vi "Calculate_Error_Rate.vi"(6 "Dataset(In1D_Out1D)":T1, 11 "Predictions":sgl[][](array[numeric])) -> (3 "Numeric":dbl)   [LabVIEW 2020]
uses:
  <vilib>/Ngene/DeepLTK/Toolkit/NN_Data/API/DataSet_Types/NN_DataSet(In1D_Out1D).ctl
  <vilib>/Ngene/DeepLTK/Toolkit/NN_Data/API/DataRef_Types/NN_Data_ref(2D_SGL).ctl
  <vilib>/Ngene/DeepLTK/Toolkit/NN_Data/API/DataRef_Types/NN_Data_ref(1D_I32).ctl
  <vilib>/Ngene/DeepLTK/Toolkit/NN_Data/subVIs/Get_Data_Vals/NN_Data_Get_ValByRef(2D_SGL).vi
  <vilib>/Ngene/DeepLTK/Toolkit/Deep_Learning_Toolkit_by_Ngene.lvlib
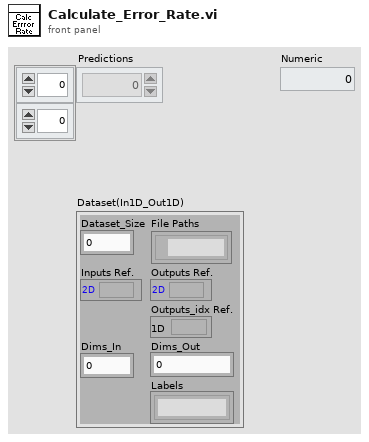
[diagram p1: front panel]
types:
  T1 = typedef "Deep_Learning_Toolkit_by_Ngene.lvlib/NN_DataSet(In1D_Out1D).ctl" = cluster{"Inputs Ref.":T2, "Outputs Ref.":T2, "Dims_In":i32, "Dataset_Size":i32, "Outputs_idx Ref.":T3, "Dims_Out":i32, "Labels":string[], "File Paths":path[]}
  T2 = typedef "Deep_Learning_Toolkit_by_Ngene.lvlib/NN_Data_ref(2D_SGL).ctl" = refnum<data-value>
  T3 = typedef "Deep_Learning_Toolkit_by_Ngene.lvlib/NN_Data_ref(1D_I32).ctl" = refnum<data-value>
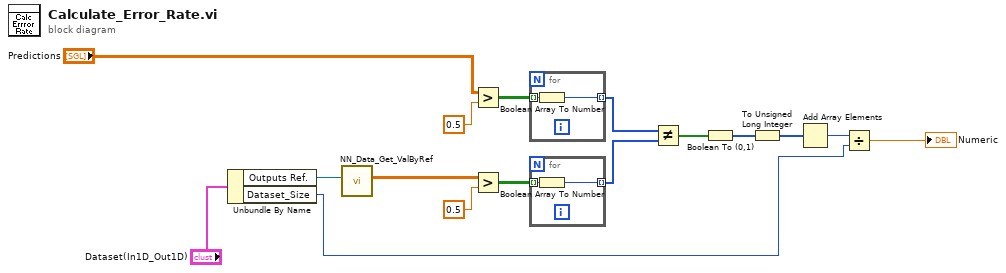
[diagram p0: block diagram]
diagram:
  n1 = Unbundle By Name("Dataset(In1D_Out1D)") -> ("Outputs Ref."=w2:T2, "Dataset_Size"=w14:i32)
  n2 = call-poly <vilib>:"NN_Data_Get_ValByRef.vi"("DVR(2D_SGL)"=w2) -> ("Value(2D_SGL)"=w12:sgl[][])  [unwired: 7 in, 1 out]
  n3 = Greater?(x="Predictions", y=sgl 0.5) -> (0:w5:bool[][])
  n4 = Greater?(x=w12, y=sgl 0.5) -> (0:w4:bool[][])
  n5 = for {
    tunnel: w5 -> [w18] mode=indexing
    tunnel: [w17] -> w8 mode=indexing
    n6 = Boolean Array To Number(Boolean array=w18) -> (number=w17:u8)
  }
  n7 = for {
    tunnel: w4 -> [w20] mode=indexing
    tunnel: [w19] -> w9 mode=indexing
    n8 = Boolean Array To Number(Boolean array=w20) -> (number=w19:u8)
  }
  n9 = Not Equal?(x=w8, y=w9) -> (x != y?=w10:bool[])
  n10 = Boolean To (0,1)(Boolean=w10) -> (0, 1=w11:i16[])
  n11 = To Unsigned Long Integer(number=w11) -> (unsigned 32bit integer=w15:u32[])
  n12 = Add Array Elements(numeric array=w15) -> (sum=w13:u32)
  n13 = Divide(x=w13, y=w14) -> (x/y=→"Numeric":dbl)
